vi "Generate Waveform.vi"(0 "Multitone in":refnum<class "SV Multitone.lvclass">, 5 "template waveform":waveform(dbl), 9 "samples":i32, 11 "error in (no error)":errorcluster) -> (4 "Multitone out":refnum<class "SV Multitone.lvclass">, 6 "output waveform":waveform(dbl), 10 "samples":i32, 15 "error out":errorcluster)   [LabVIEW 2017, in "SV Multitone.lvclass"]
uses:
  <vilib>/addons/_NISVFA/_Generation/Signal Generation/SV Multitone/SV Multitone.lvclass
  C:/Program Files (x86)/National Instruments/LabVIEW 2017/vi.lib/addons/_NISVFA/_Generation/Signal Generation/SV Signal/SV Signal.lvclass
  <vilib>/addons/_NISVFA/_Generation/Signal Generation/SV Multitone/SV Multitone.lvclass/SV Multitone.ctl
  <vilib>/addons/_NISVFA/_Generation/Signal Generation/SV Signal/sv_Signal State Attribute.ctl
  <vilib>/addons/_NISVFA/_Generation/Signal Generation/SV Signal/Read Sample Rate.vi
  <vilib>/Analysis/NI_AALBase.lvlib
  <vilib>/addons/_NISVFA/_Generation/Signal Generation/SV Signal/SV Signal.lvclass
  <vilib>/measure/NI_MABase.lvlib
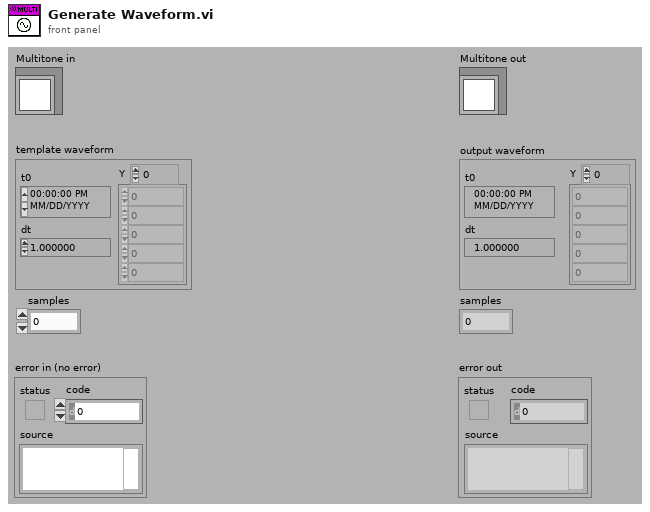
[diagram p1: front panel]
types:
  T1 = typedef "SV Signal.lvclass/sv_Signal State Attribute.ctl" = string
  T2 = typedef "SV Signal.lvclass/sv_System Timing Model.ctl" = i64
  T3 = typedef "SV Signal.lvclass/sv_Generation State.ctl" = enum16{"Idle", "Ramp Up", "Pre-Measurement Settling", "Measurement", "Post-Measurement Settling", "Discrete Sweep Transition", "Ramp Down", "Update"}
  T4 = cluster{"system timing model":T2, "state":cluster{"RESET":bool, "generator timestamp":timestamp, "elapsed seconds":dbl, "elapsed samples":u64, "generation state":T3, "time offset at state":dbl, "samples generated at state":u64, "signal state":variant}, "duration of state":dbl, "samples remaining at state":i32}
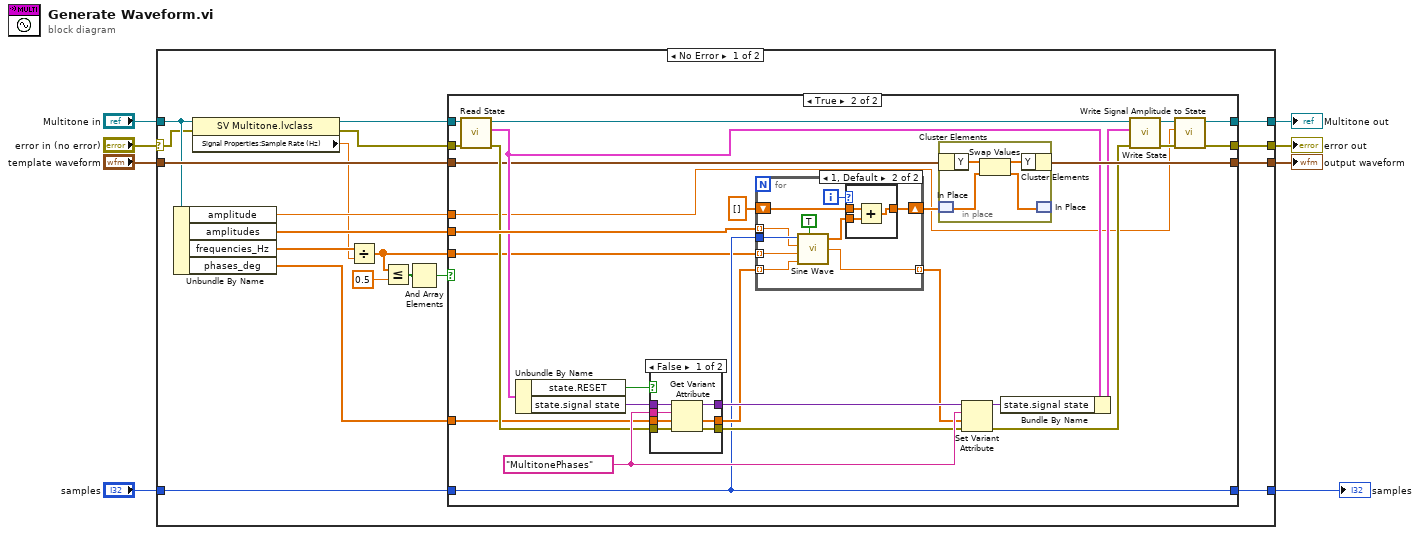
[diagram p0: block diagram]
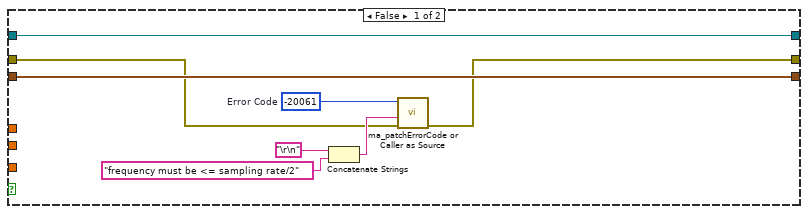
[diagram p2: hidden frame]
diagram:
  n1 = case shown="No Error" "error in (no error)" {
    selector: "error in (no error)" -> [w19 w94]
    tunnel: [w22 w94] -> w7
    tunnel: [w23 w93] -> w5
    tunnel: "Multitone in" -> [w20 w93]
    tunnel: [w27 w92] -> w4
    tunnel: [w13 _] -> w3
    tunnel: "samples" -> [w26 _]
    tunnel: "template waveform" -> [w24 w92]
    frame No Error {
      n2 = Unbundle By Name(w20) -> ("amplitude"=w21:dbl, "amplitudes"=w25:dbl[], "frequencies_Hz"=w17:dbl[], "phases_deg"=w14:dbl[])
      n3 = property class="SV Multitone.lvclass"(reference=w20, error in=w19) -> (reference out=w15:refnum<class "SV Multitone.lvclass">, error out=w18:errorcluster, "Signal Properties:Sample Rate (Hz)"=w16:dbl)
      n4 = Divide(x=w17, y=w16) -> (x/y=w11:dbl[])
      n5 = Less Or Equal?(x=w11, y=0.5) -> (x <= y?=w9:bool[])
      n6 = And Array Elements(Boolean array=w9) -> (logical AND=w10:bool)
      n7 = case shown="True" w10 {
        tunnel: [w34 w63] -> w27
        tunnel: w26 -> [_ w40]
        tunnel: w25 -> [_ w62]
        tunnel: w24 -> [w34 w48]
        tunnel: [w35 w38] -> w23
        tunnel: [w28 w37] -> w22
        tunnel: w21 -> [_ w45]
        tunnel: w18 -> [w29 w44]
        tunnel: w11 -> [_ w39]
        tunnel: w15 -> [w35 w43]
        tunnel: w14 -> [_ w41]
        tunnel: [_ w40] -> w13
        frame False {
          w30 = -20061  # Error Code
          n8 = Concatenate Strings("\r\n", "frequency must be <= sampling rate/2" ("freq error message")) -> (w33:string)
          n9 = call <vilib>:"ma_patchErrorCode or Caller as Source.vi"("error in (no error)"=w29, "string to append to source"=w33, "error code"=w30) -> ("error out"=w28:errorcluster)  [unwired: 8 in]
        }
        frame True {
          w58 = T1 "MultitonePhases" ("name")
          n10 = call <vilib>:"Read State.vi"("error in (no error)"=w44, "signal configuration"=w43) -> ("error out"=w53:errorcluster, "generator state"=w49:T4, "signal configuration"=w42:refnum<class "SV Multitone.lvclass">)  [unwired: 7 in]
          n11 = Unbundle By Name(w49) -> ("state.RESET"=w36:bool, "state.signal state"=w61:variant)
          n12 = case shown="False" w36 {
            tunnel: w61 -> [w70 w73]
            tunnel: w41 -> [w69 w72]
            tunnel: [w68 w73] -> w60
            tunnel: w58 -> [w67 _]
            tunnel: [w66 w72] -> w56
            tunnel: w53 -> [w65 w71]
            tunnel: [w64 w71] -> w52
            frame False {
              n13 = Get Variant Attribute(Variant=w70, name=w67, default value (empty Variant)=w69, error in=w65) -> (duplicate Variant=w68:variant, value=w66:dbl[], error out=w64:errorcluster)  [unwired: 1 out]
            }
            frame True {
            }
          }
          n14 = for {
            tunnel: w40 -> [w83]
            tunnel: w62 -> [w81] mode=indexing
            tunnel: [w80] -> w57 mode=indexing
            tunnel: w56 -> [w79] mode=indexing
            shift-right: [w76] -> w54
            shift-left: dbl[] [] ("sine wave") -> [w75]
            tunnel: w39 -> [w74] mode=indexing
            i -> [w78]
            n15 = call <vilib>:"Sine Wave.vi"("samples"=w83, "amplitude"=w81, "frequency"=w74, "phase in"=w79, "reset phase"=TRUE ("coerce frequencies?")) -> ("sine wave"=w77:dbl[], "phase out"=w80:dbl)  [unwired: 1 out]
            n16 = case shown="1, Default" w78 {
              tunnel: w77 -> [w84 w87]
              tunnel: [w84 w86] -> w76
              tunnel: w75 -> [_ w85]
              frame 0 {
              }
              frame 1, Default {
                n17 = Add(x=w85, y=w87) -> (x+y=w86:dbl[])
              }
            }
          }
          n18 = in-place {
            n19 = in-place-cluster #1(w48) -> ("Y"=w91:dbl[])
            n20 = in-place-match #2(w54) -> (w90:dbl[])
            n21 = Swap Values(12:w91, 14:w90) -> (1:w89:dbl[], 3:w88:dbl[])  [unwired: 1 in]
            n22 = in-place-cluster #1("Y"=w89) -> (w63:waveform(dbl))
            n23 = in-place-match #2(w88) -> ()  [unwired: 1 out]
          }
          n24 = Set Variant Attribute(Variant=w60, name=w58, value=w57, error in=w52) -> (Variant out=w59:variant, error out=w51:errorcluster)  [unwired: 1 out]
          n25 = Bundle By Name(cluster=w49, "state.signal state"=w59) -> (w50:T4)
          n26 = call <vilib>:"Write State.vi"("error in (no error)"=w51, "generator state"=w50, "signal configuration"=w42) -> ("error out"=w46:errorcluster, "signal configuration"=w47:refnum<class "SV Multitone.lvclass">)  [unwired: 7 in]
          n27 = call <vilib>:"Write Signal Amplitude to State.vi"("error in (no error)"=w46, "amplitude"=w45, "SV Signal in"=w47) -> ("error out"=w37:errorcluster, "SV Signal out"=w38:refnum<class "SV Multitone.lvclass">)  [unwired: 7 in]
        }
      }
    }
    frame Error {
    }
  }
  "error out" <- w7
  "Multitone out" <- w5
  "output waveform" <- w4
  "samples" <- w3
